vi "DrawBorder.vi"(9 "display in":picture, 11 "Cell in":refnum<class "Cell.lvclass">) -> (1 "display out":picture, 3 "Cell out":refnum<class "Cell.lvclass">)   [LabVIEW 2021, in "Cell.lvclass"]
uses:
  Cell.lvclass
  Cell.lvclass/Cell.ctl
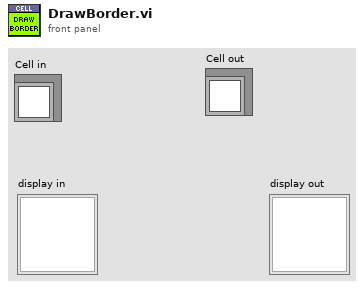
[diagram p1: front panel]
types:
  T1 = cluster{"Width":i16, "Style":enum32{"Solid", "Dash", "Dot", "DashDot", "DashDotDot"}}
  T2 = cluster{"left":i16, "top":i16, "right":i16, "bottom":i16}
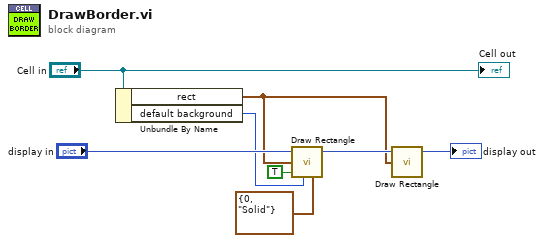
[diagram p0: block diagram]
diagram:
  n1 = Unbundle By Name("Cell in") -> ("rect"=w2:T2, "default background"=w5:u32)
  n2 = call <vilib>:"Draw Rectangle.vi"("picture"="display in", "rect"=w2, "fill?(F)"=TRUE, "color(black)"=w5, "pen"=T1 {"Width"=0, "Style"=enum."Solid"}) -> ("new picture"=w3:picture)  [unwired: 4 in]
  n3 = call <vilib>:"Draw Rectangle.vi"("picture"=w3, "rect"=w2) -> ("new picture"=→"display out":picture)  [unwired: 7 in]
  "Cell out" <- "Cell in"
